vi "SparsePCA.vi"(8 "error in":errorcluster) -> (0 "error out":errorcluster, 3 "out":refnum<class "SparsePCA.lvclass">)   [LabVIEW 2020]
doc: "Sparse Principal Components Analysis (SparsePCA).\n\n Finds the set of sparse components that can optimally reconstruct\n the data. The amount of sparseness is controllable by the coefficient\n of the L1 penalty, given by the parameter alpha.\n\n Read more in the :ref:`User Guide <SparsePCA>`.\n\n Parameters\n ----------\n n_components : int, default=None\n Number of sparse atoms to extract.\n\n alpha : float, default=1\n Sparsity controlling parameter. Higher values lead to sparser\n components.\n\n ridge_alpha : float, default=0.01\n Amount of ridge shrinkage to apply in order to improve\n conditioning when calling the transform method.\n\n max_iter : int, default=1000\n Maximum number of iterations to perform.\n\n tol : float, default=1e-8\n Tolerance for the stopping condition.\n\n method : {'lars', 'cd'}, default='lars'\n lars: uses the least angle regression method to solve the lasso problem\n (linear_model.lars_path)\n cd: uses the coordinate descent method to compute the\n Lasso solution (linear_model.Lasso). Lars will be faster if\n the estimated components are sparse.\n\n n_jobs : int, default=None\n Number of parallel jobs to run.\n ``None`` means 1 unless in a :obj:`joblib.parallel_backend` context.\n ``-1`` means using all processors. See :term:`Glossary <n_jobs>`\n for more details.\n\n U_init : ndarray of shape (n_samples, n_components), default=None\n Initial values for the loadings for warm restart scenarios. Only used\n if `U_init` and `V_init` are not None.\n\n V_init : ndarray of shape (n_components, n_features), default=None\n Initial values for the components for warm restart scenarios. Only used\n if `U_init` and `V_init` are not None.\n\n verbose : int or bool, default=False\n Controls the verbosity; the higher, the more messages. Defaults to 0.\n\n random_state : int, RandomState instance or None, default=None\n Used during dictionary learning. Pass an int for reproducible results\n across multiple function calls.\n See :term:`Glossary <random_state>`.\n\n Attributes\n ----------\n components_ : ndarray of shape (n_components, n_features)\n Sparse components extracted from the data.\n\n error_ : ndarray\n Vector of errors at each iteration.\n\n n_components_ : int\n Estimated number of components.\n\n .. versionadded:: 0.23\n\n n_iter_ : int\n Number of iterations run.\n\n mean_ : ndarray of shape (n_features,)\n Per-feature empirical mean, estimated from the training set.\n Equal to ``X.mean(axis=0)``.\n\n \nAvailable methods:\nFit\nFit Transform\nTransform\nGet Attributes\nGet Params\nSet Params"
uses:
  SparsePCA.lvclass
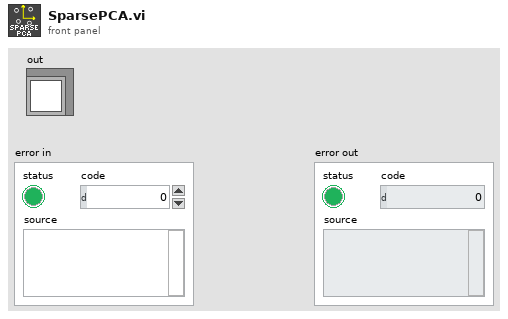
[diagram p1: front panel]
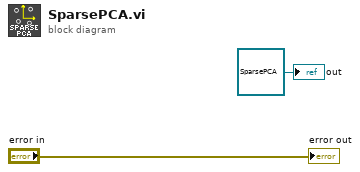
[diagram p0: block diagram]
diagram:
  "out" <- refnum<class "SparsePCA.lvclass"> refnum ("model")
  "error out" <- "error in"
